vi "Get Font Color.vi"(11 "is valid?":bool) -> (3 "font color":u32)   [LabVIEW 2021, in "MeasurementClient Editor.lvlib"]
uses:
  MeasurementClient Editor.lvlib
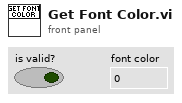
[diagram p1: front panel]
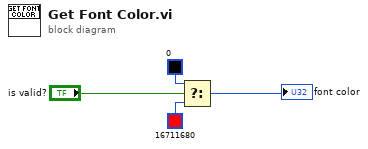
[diagram p0: block diagram]
diagram:
  n1 = Select(t=u32 0 ("Active Cell:Cell Font:Color"), s="is valid?", f=u32 16711680 ("Active Cell:Cell Font:Color")) -> (s? t:f=→"font color":u32)
